vi "String.Look Up from List, with Mask.vi"(8 "Str List":string[](array[string])=["AUAK820110D5", "AUAK820110D6", "AUAK820110D7", "AUAK820110D8"], 9 "Mask Justification(F=Right/T=Left)":bool, 10 "Mask":string="000000011111", 11 "Str":string="AUAK8201\t10D6") -> (3 "Is Match":bool)   [LabVIEW 2018]
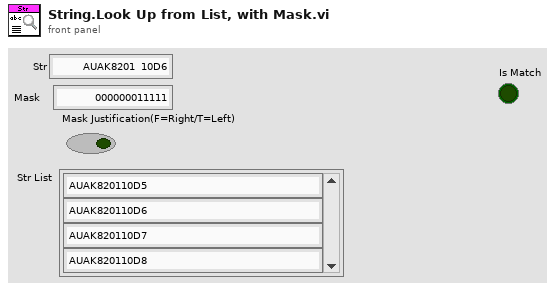
[diagram p1: front panel]
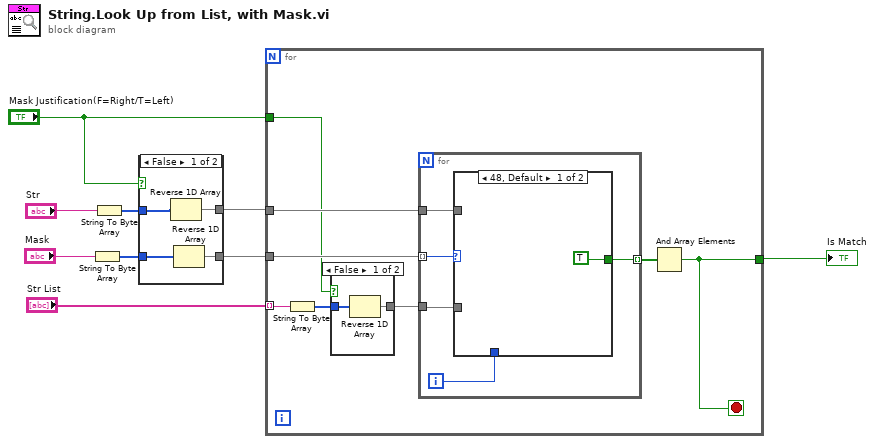
[diagram p0: block diagram]
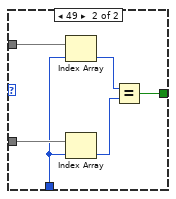
[diagram p4: hidden frame]
diagram:
  n1 = String To Byte Array(string="Mask") -> (unsigned byte array=w3:u8[])
  n2 = String To Byte Array(string="Str") -> (unsigned byte array=w5:u8[])
  n3 = case shown="False" "Mask Justification(F=Right/T=Left)" {
    tunnel: w5 -> [w13 w15]
    tunnel: [w12 w15] -> w4
    tunnel: w3 -> [w11 w14]
    tunnel: [w10 w14] -> w2
    frame False {
      n4 = Reverse 1D Array(array=w13) -> (reversed array=w12:u8[])
      n5 = Reverse 1D Array(array=w11) -> (reversed array=w10:u8[])
    }
    frame True {
    }
  }
  n6 = for {
    tunnel: "Str List" -> [w23] mode=indexing
    tunnel: w4 -> [w22]
    tunnel: w2 -> [w21]
    tunnel: [w19] -> w6
    tunnel: "Mask Justification(F=Right/T=Left)" -> [w16]
    stop <- w19 stop-if-true
    n7 = String To Byte Array(string=w23) -> (unsigned byte array=w18:u8[])
    n8 = case shown="False" w16 {
      tunnel: w18 -> [w25 w26]
      tunnel: [w24 w26] -> w17
      frame False {
        n9 = Reverse 1D Array(array=w25) -> (reversed array=w24:u8[])
      }
      frame True {
      }
    }
    n10 = for {
      tunnel: w22 -> [w31]
      tunnel: w21 -> [w28] mode=indexing
      tunnel: w17 -> [w30]
      tunnel: [w27] -> w20 mode=indexing
      i -> [w29]
      n11 = case shown="48, Default" w28 {
        tunnel: w31 -> [_ w38]
        tunnel: w30 -> [_ w37]
        tunnel: w29 -> [_ w36]
        tunnel: [TRUE w33] -> w27
        frame 48, Default {
        }
        frame 49 {
          n12 = Index Array(array=w38, index=w36) -> (element=w35:u8)
          n13 = Index Array(array=w37, index=w36) -> (element=w34:u8)
          n14 = Equal?(x=w35, y=w34) -> (x = y?=w33:bool)
        }
      }
    }
    n15 = And Array Elements(Boolean array=w20) -> (logical AND=w19:bool)
  }
  "Is Match" <- w6
